vi "test_Format Time (Good Time).vi"(8 "error in (no error)":errorcluster, 11 "TestCase in":refnum<class "Test Simple Layout.lvclass">) -> (0 "error out":errorcluster, 3 "TestCase out":refnum<class "Test Simple Layout.lvclass">)   [LabVIEW 2019, in "Test Simple Layout.lvclass"]
uses:
  Test Simple Layout.lvclass
  C:/Program Files/National Instruments/LabVIEW 2024/vi.lib/Astemes/LUnit/Test Case.lvclass
  <vilib>/Astemes/LUnit/Test Case.lvclass/Test Case.ctl
  567c9f1c-3be0-42dd-86f5-ffc451e7245c.vi
  <vilib>/Astemes/LUnit/Core/LUnit Test Case/Private/Append Pass Result.vi
  <vilib>/Astemes/LUnit/Core/LUnit Test Case/Private/Append Fail Result.vi
  567c9f1c-3be0-42dd-86f5-ffc451e7245c.vi/9c5d11cd-9439-4240-a1ee-d9baace9c924.vi
  <vilib>/Astemes/LUnit/Core/LUnit Test Case/Private/Run In UI.vi
  <vilib>/Utility/error.llb/Clear Errors.vi
  Layouts/Layout.lvclass
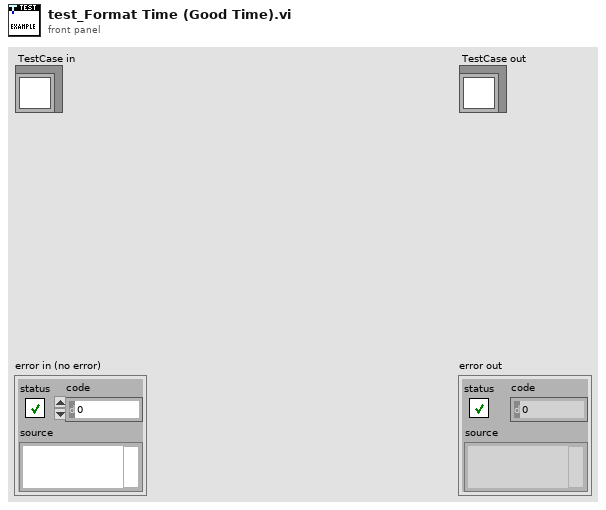
[diagram p1: front panel]
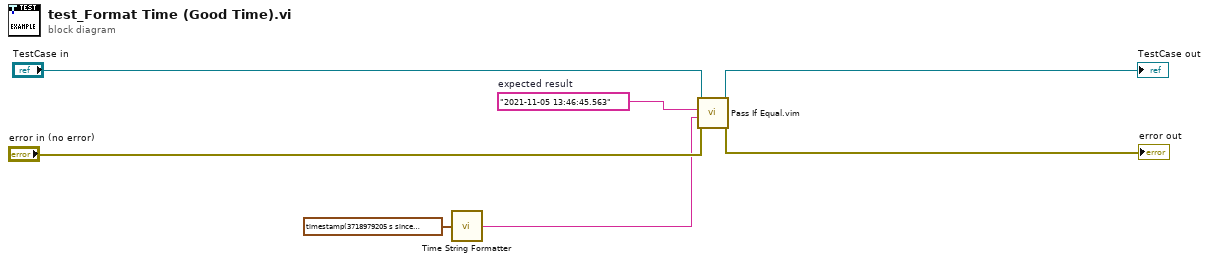
[diagram p0: block diagram]
diagram:
  w3 = "2021-11-05 13:46:45.563"  # expected result
  n1 = call "Time String Formatter.vi"("Time"=timestamp(3718979205.5636735 s since 1904-01-01)) -> ("Time string"=w2:string)
  n2 = call "Pass If Equal.vim"("error in (no error)"="error in (no error)", "Actual"=w2, "Expected"=w3, "LUnit Test Case In"="TestCase in") -> ("error out"=→"error out":errorcluster, "LUnit Test Case Out"=→"TestCase out":refnum<class "Test Simple Layout.lvclass">)  [unwired: 6 in]
